vi "Login.vi"(1 "Passwords":string[](array[string]), 2 "Password":string, 3 "Usernames":string[](array[string]), 4 "Username":string) -> (0 "Login Attempts":i8)   [LabVIEW 2017]
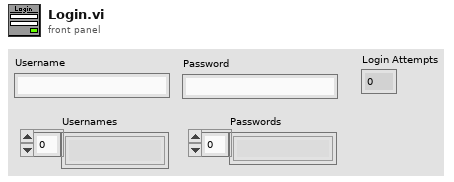
[diagram p1: front panel]
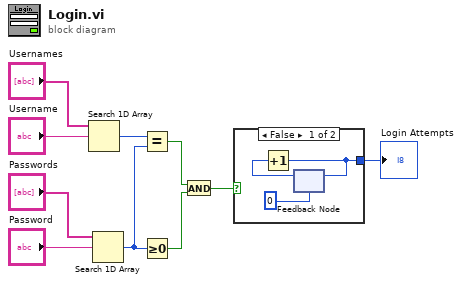
[diagram p0: block diagram]
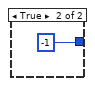
[diagram p2: hidden frame]
diagram:
  n1 = Search 1D Array(1D array="Usernames", element="Username") -> (index of element=w8:i32)  [unwired: 1 in]
  n2 = Search 1D Array(1D array="Passwords", element="Password") -> (index of element=w9:i32)  [unwired: 1 in]
  n3 = Equal?(x=w8, y=w9) -> (x = y?=w6:bool)
  n4 = Greater Or Equal To 0?(x=w9) -> (x >= 0?=w7:bool)
  n5 = And(x=w6, y=w7) -> (x .and. y?=w3:bool)
  n6 = case shown="False" w3 {
    tunnel: [w11 -1] -> w4
    frame False {
      n7 = feedback #1(0) -> (w11:i32)
      n8 = Increment(x=w11) -> (x+1=w13:i32)
      n9 = feedback-in #1(w13) -> ()
    }
    frame True {
    }
  }
  "Login Attempts" <- w4
